vi "DecodeCloseReason.vi"(10 "Data":string) -> (1 "Reason":string, 2 "Status Code":T1=1000 items=["Normal Closure"=1000, "Going Away"=1001, "Protocol Error"=1002, "Wrong Data Type"=1003, "Reserved 1004"=1004, "Reserved 1005"=1005, "Reserved 1006"=1006, "Non Consistent Data Type"=1007, "Policy Violation"=1008, "Message Too Big"=1009, "Extensions Negotiation Error"=1010, "Unexpected Condition"=1011, "Reserved 1015"=1015], 3 "Close Reason Given":bool)   [LabVIEW 2016, in "WebSockets.lvlib"]
uses:
  WebSockets.lvlib
  StatusCode.ctl
panel:
  out "error out":errorcluster
  in  "error in (no error)":errorcluster
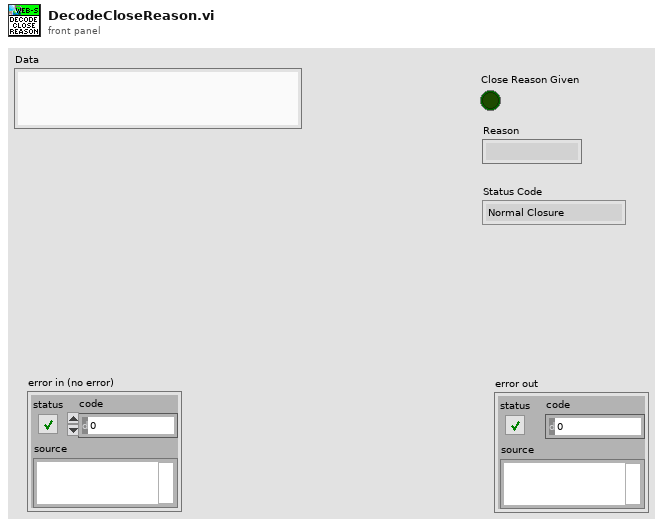
[diagram p1: front panel]
types:
  T1 = typedef "WebSockets.lvlib/StatusCode.ctl" = u16
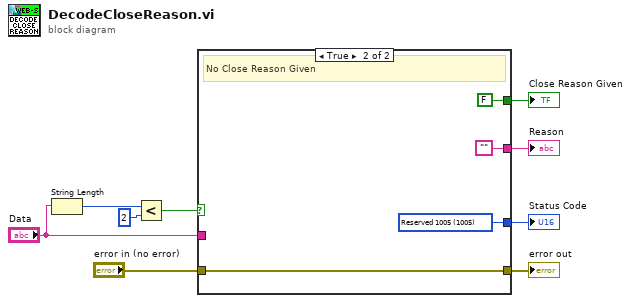
[diagram p0: block diagram]
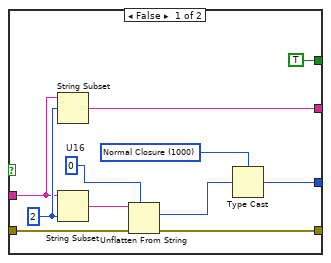
[diagram p2: hidden frame]
diagram:
  n1 = String Length(string="Data") -> (length=w9:i32)
  n2 = Less?(x=w9, y=2) -> (x < y?=w7:bool)
  n3 = case shown="True" w7 {
    tunnel: [TRUE ("No Close Reason Given") FALSE ("No Close Reason Given")] -> w6
    tunnel: "Data" -> [w18 _]
    tunnel: [w17 ""] -> w5
    tunnel: [w14 w23] -> w4
    tunnel: "error in (no error)" -> [w13 w23]
    tunnel: [w10 w21] -> w2
    frame False {
      w11 = T1 1000 items=["Normal Closure"=1000, "Going Away"=1001, "Protocol Error"=1002, "Wrong Data Type"=1003, "Reserved 1004"=1004, "Reserved 1005"=1005, "Reserved 1006"=1006, "Non Consistent Data Type"=1007, "Policy Violation"=1008, "Message Too Big"=1009, "Extensions Negotiation Error"=1010, "Unexpected Condition"=1011, "Reserved 1015"=1015] ("Status Code")
      w15 = u16 0  # U16
      w19 = 2 ("length (rest)")
      n4 = String Subset(string=w18, offset (0)=w19) -> (substring=w17:string)  [unwired: 1 in]
      n5 = String Subset(string=w18, length (rest)=w19) -> (substring=w16:string)  [unwired: 1 in]
      n6 = Unflatten From String(type=w15, binary string=w16, error in (no error)=w13) -> (value=w12:u16, error out=w14:errorcluster)  [unwired: 2 in, 1 out]
      n7 = Type Cast(type=w11, x=w12) -> (*(type *) &x=w10:T1)
    }
    frame True {
      w21 = T1 1005 items=["Normal Closure"=1000, "Going Away"=1001, "Protocol Error"=1002, "Wrong Data Type"=1003, "Reserved 1004"=1004, "Reserved 1005"=1005, "Reserved 1006"=1006, "Non Consistent Data Type"=1007, "Policy Violation"=1008, "Message Too Big"=1009, "Extensions Negotiation Error"=1010, "Unexpected Condition"=1011, "Reserved 1015"=1015] ("Status Code")
      # "No Close Reason Given"
    }
  }
  "Close Reason Given" <- w6
  "Reason" <- w5
  "error out" <- w4
  "Status Code" <- w2
